vi "Obtain Components Ref.vi"(8 "error in (no error)":errorcluster, 11 "Item Ref in":T1 format="%.0x") -> (0 "error out":errorcluster, 1 "created new?":bool, 2 "comps notifier":refnum<notifier>, 3 "Item Ref out":T1 format="%.0x")   [LabVIEW 2017, in "DSF System Explorer.lvlib"]
uses:
  DSF System Explorer.lvlib
  <vilib>/NI Veristand/Custom Device API/Custom Device Item Ref.ctl
  DSF Core.lvlibp/Classes/Component/Component.lvclass
  <vilib>/NI Veristand/Custom Device API/Custom Device API.lvlib
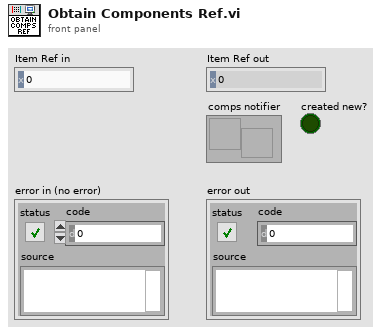
[diagram p1: front panel]
types:
  T1 = typedef "Custom Device API.lvlib/Custom Device Item Ref.ctl" = u64
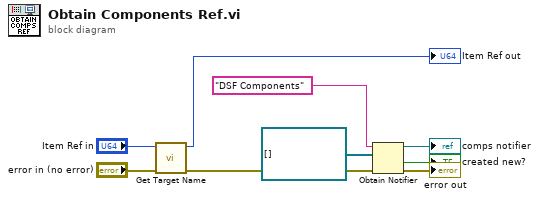
[diagram p0: block diagram]
diagram:
  n1 = call "Get Target Name.vi"("error in (no error)"="error in (no error)", "Node Ptr"="Item Ref in") -> ("error out"=w7:errorcluster, "Item Ref out"=→"Item Ref out":T1)  [unwired: 6 in, 2 out]
  n2 = Obtain Notifier(name (unnamed)="DSF Components", notification data type=refnum<class "Component.lvclass">[] [] ("Components"), error in (no error)=w7) -> (notifier out=→"comps notifier":refnum<notifier>, created new?=→"created new?":bool, error out=→"error out":errorcluster)  [unwired: 1 in]
